vi "test_CCDAllTests.vi"(7 "Test should pass":bool=TRUE, 8 "error in":errorcluster, 9 "tear down connection":bool=TRUE, 10 "set-up a connection":bool=TRUE, 11 "device selection":enum16{"monochromator", "CCD", "SCD"}(ring)=enum."CCD") -> (0 "error out":errorcluster, 1 "log-file path":path)   [LabVIEW 2023]
uses:
  Classes/CCD/CCD.lvclass
  C:/Projects/Horiba/horiba-labview-sdk/Source/Classes/GenericDevice/GenericDevice.lvclass
  <vilib>/addons/_JKI Toolkits/Caraya/classes/Test/Test.lvclass
  <vilib>/Hampel Software Engineering/HSE Logger/hse-logger.lvlib
panel:
  # "Connector Pane"
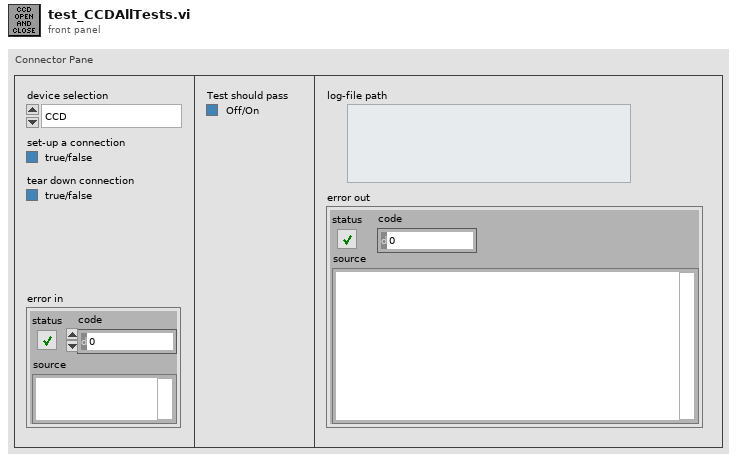
[diagram p1: front panel]
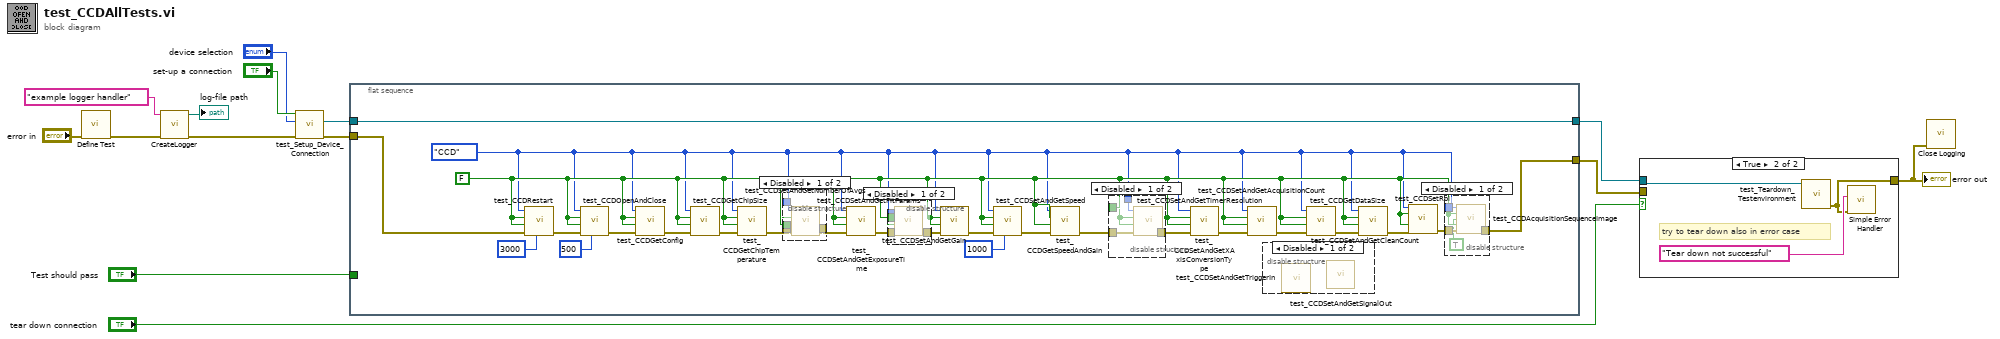
[diagram p0: block diagram]
diagram:
  n1 = call <vilib>:"Define Test.vi"("error in (no error)"="error in") -> ("error out"=w2:errorcluster)  [unwired: 9 in, 1 out]
  n2 = call "CreateLogger.vi"("error in (no error)"=w2, "Handler Name"="example logger handler") -> ("error out"=w1:errorcluster, "log-file path"=→"log-file path":path)  [unwired: 8 in]
  n3 = call "test_Setup_Device_Connection.vi"("error in (no error)"=w1, "device selection"="device selection", "set-up a connection"="set-up a connection") -> ("error out"=w6:errorcluster, "CCD.lvclass"=w7:refnum<class "CCD.lvclass">)  [unwired: 5 in, 2 out]
  n4 = flat-sequence {
    tunnel: w6 -> [w25]
    tunnel: w7 -> [w33]
    tunnel: [w20] -> w11
    tunnel: "Test should pass" -> [_]
    tunnel: [w33] -> w10
    frame #0 {
      w17 = enum16{"monochromator", "CCD", "SCD"}."CCD" ("device selection")
      w18 = FALSE
      n5 = call "test_CCDRestart.vi"("Delay between send and receive [ms]"=3000, "error in"=w25, "tear down connection"=w18, "set-up a connection"=w18, "device selection"=w17) -> ("error out"=w26:errorcluster)  [unwired: 6 in]
      n6 = call "test_CCDOpenAndClose.vi"("Delay between send and receive [ms]"=500, "error in"=w26, "tear down connection"=w18, "set-up a connection"=w18, "device selection"=w17) -> ("error out"=w19:errorcluster)  [unwired: 6 in]
      n7 = call "test_CCDGetConfig.vi"("error in"=w19, "tear down connection"=w18, "set-up a connection"=w18, "device selection"=w17) -> ("error out"=w16:errorcluster)  [unwired: 7 in]
      n8 = call "test_CCDGetChipSize.vi"("error in"=w16, "tear down connection"=w18, "set-up a connection"=w18, "device selection"=w17) -> ("error out"=w39:errorcluster)  [unwired: 7 in]
      n9 = call "test_CCDGetChipTemperature.vi"("error in"=w39, "tear down connection"=w18, "set-up a connection"=w18, "device selection"=w17) -> ("error out"=w31:errorcluster)  [unwired: 7 in]
      n10 = disable-structure shown="Disabled" {
        disable-tunnel: w31 -> [w59 w60]
        disable-tunnel: [w58 w60] -> w30
        disable-tunnel: w17 -> [w57 _]
        disable-tunnel: w18 -> [w56 _]
        frame Disabled {
          n11 = call "test_CCDSetAndGetNumberOfAvgs.vi"("error in"=w59, "tear down connection"=w56, "set-up a connection"=w56, "device selection"=w57) -> ("error out"=w58:errorcluster)  [unwired: 7 in]
        }
        frame Enabled {
        }
      }
      n12 = call "test_CCDSetAndGetExposureTime.vi"("error in"=w30, "tear down connection"=w18, "set-up a connection"=w18, "device selection"=w17) -> ("error out"=w38:errorcluster)  [unwired: 7 in]
      n13 = disable-structure shown="Disabled" {
        disable-tunnel: w38 -> [w54 w55]
        disable-tunnel: [w53 w55] -> w37
        disable-tunnel: w17 -> [w52 _]
        disable-tunnel: w18 -> [w51 _]
        frame Disabled {
          n14 = call "test_CCDSetAndGetFitParams.vi"("error in"=w54, "tear down connection"=w51, "set-up a connection"=w51, "device selection"=w52) -> ("error out"=w53:errorcluster)  [unwired: 7 in]
        }
        frame Enabled {
        }
      }
      n15 = call "test_CCDSetAndGetGain.vi"("error in"=w37, "tear down connection"=w18, "set-up a connection"=w18, "device selection"=w17) -> ("error out"=w32:errorcluster)  [unwired: 7 in]
      n16 = call "test_CCDSetAndGetSpeed.vi"("Delay between send and receive [ms]"=1000, "error in"=w32, "tear down connection"=w18, "set-up a connection"=w18, "device selection"=w17) -> ("error out"=w23:errorcluster)  [unwired: 6 in]
      n17 = call "test_CCDGetSpeedAndGain.vi"("error in"=w23, "tear down connection"=w18, "set-up a connection"=w18, "device selection"=w17) -> ("error out"=w15:errorcluster)  [unwired: 4 in, 3 out]
      n18 = disable-structure shown="Disabled" {
        disable-tunnel: [w49 w50] -> w36
        disable-tunnel: w15 -> [w48 w50]
        disable-tunnel: w18 -> [w47 _]
        disable-tunnel: w17 -> [w46 _]
        frame Disabled {
          n19 = call "test_CCDSetAndGetTimerResolution.vi"("error in"=w48, "tear down connection"=w47, "set-up a connection"=w47, "device selection"=w46) -> ("error out"=w49:errorcluster)  [unwired: 7 in]
        }
        frame Enabled {
        }
      }
      n20 = call "test_CCDSetAndGetXAxisConversionType.vi"("error in"=w36, "tear down connection"=w18, "set-up a connection"=w18, "device selection"=w17) -> ("error out"=w35:errorcluster)  [unwired: 7 in]
      n21 = call "test_CCDSetAndGetAcquisitionCount.vi"("error in"=w35, "tear down connection"=w18, "set-up a connection"=w18, "device selection"=w17) -> ("error out"=w34:errorcluster)  [unwired: 7 in]
      n22 = disable-structure shown="Disabled" {
        frame Disabled {
          n23 = call "test_CCDSetAndGetTriggerIn.vi"() -> ()  [unwired: 11 in, 1 out]
          n24 = call <vilib>:"test_CCDSetAndGetSignalOut.vi"() -> ()  [unwired: 11 in, 1 out]
        }
        frame Enabled {
        }
      }
      n25 = call "test_CCDSetAndGetCleanCount.vi"("error in"=w34, "tear down connection"=w18, "set-up a connection"=w18, "device selection"=w17) -> ("error out"=w29:errorcluster)  [unwired: 7 in]
      n26 = call "test_CCDGetDataSize.vi"("error in"=w29, "tear down connection"=w18, "set-up a connection"=w18, "device selection"=w17) -> ("error out"=w22:errorcluster)  [unwired: 7 in]
      n27 = call "test_CCDSetRoi.vi"("device selection"=w17, "set-up a connection"=w18, "tear down connection"=w18, "error in"=w22) -> ("error out"=w21:errorcluster)  [unwired: 10 in, 1 out]
      n28 = disable-structure shown="Disabled" {
        disable-tunnel: w21 -> [w44 w45]
        disable-tunnel: [w43 w45] -> w20
        disable-tunnel: w18 -> [w42 _]
        disable-tunnel: w17 -> [w41 _]
        frame Disabled {
          n29 = call "test_CCDAcquisitionSequenceImage.vi"("device selection"=w41, "set-up a connection"=w42, "set 3 ROIs / set 1 ROI"=TRUE, "tear down connection"=w42, "error in"=w44) -> ("error out"=w43:errorcluster)  [unwired: 5 in, 5 out]
        }
        frame Enabled {
        }
      }
    }
  }
  n30 = case shown="True" "tear down connection" {
    tunnel: w10 -> [_ w63]
    tunnel: [w61 w62] -> w5
    tunnel: w11 -> [w61 _]
    frame False {
    }
    frame True {
      # "try to tear down also in error case"
      n31 = call "test_Teardown_Testenvironment.vi"("GenericDevice.lvclass"=w63) -> ("error out"=w62:errorcluster)  [unwired: 9 in, 1 out]
      n32 = call <vilib>:"Simple Error Handler.vi"("error source (\" \")"="Tear down not successful" ("error source (\" \")"), "error in (no error)"=w62) -> ()  [unwired: 3 in, 5 out]
    }
  }
  "error out" <- w5
  n33 = call <vilib>:"Close Logging.vi"("error in"=w5) -> ()  [unwired: 10 in, 1 out]
